vi "INTERLOCK SETTING.vi"() -> ()   [LabVIEW 2017]
uses:
  <vilib>/addons/database/Connection.llb/DB Tools Open Connec (Path).vi
  <vilib>/addons/_office/excel.llb/Excel Get Data ([str]).vi
  <vilib>/addons/_office/excel.llb/Excel Easy Table (str).vi
  <vilib>/Utility/NIReport.llb/NI_report.lvclass
  <vilib>/addons/database/NI_Database_API.lvlib
  <vilib>/addons/_office/NI_ReportGenerationToolkit.lvlib
  <vilib>/Utility/NIReport.llb/Excel/NI_Excel.lvclass
panel:
  in  "RECIPE PATH":path
  in  "EXPORT RECIPE":bool
  in  "Import Recipe":bool
  in  "table":string[][](table)
  in  "EXIT":bool
  in  "SAVE":bool
  # "PARAMETERS VALUE"
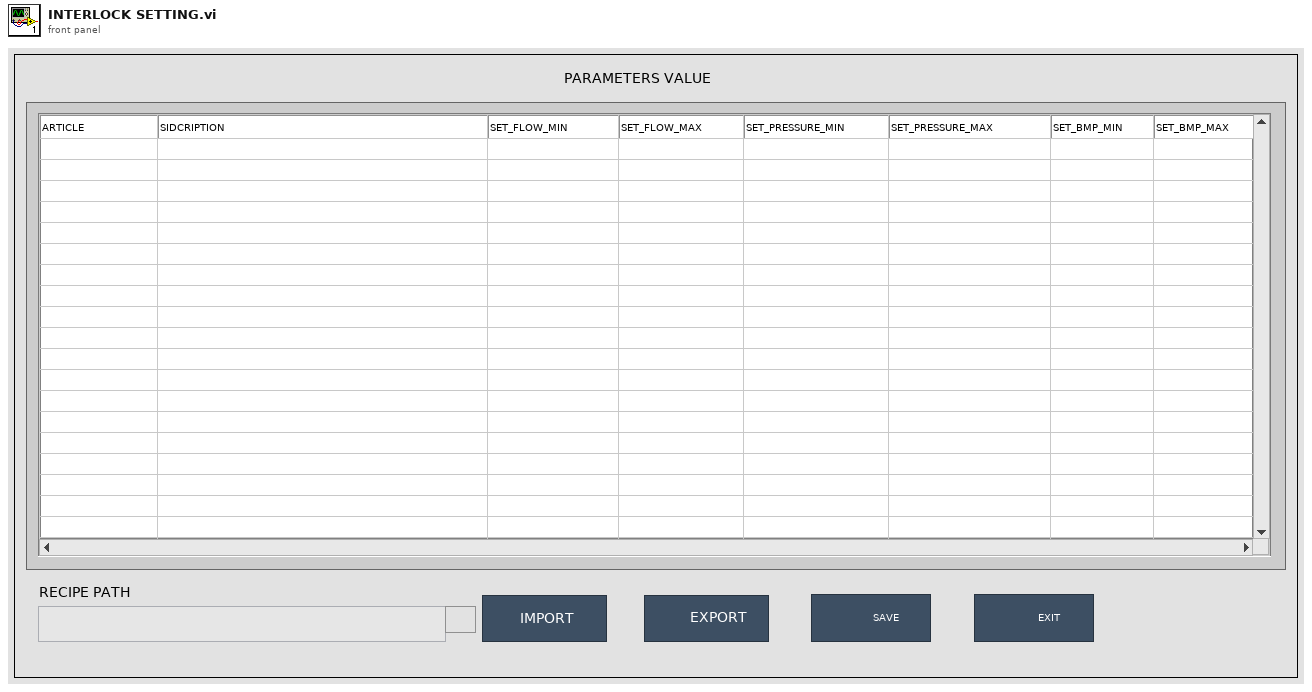
[diagram p1: front panel]
types:
  T1 = typedef "NI_Database_API.lvlib/Conn ObjectReference.ctl" = refnum<k1>
  T2 = enum16{"Standard Report", "HTML", "Word", "Excel"}
  T3 = enum16{"maximized", "minimized", "normal", "no change"}
  T4 = cluster{"table":string[], "table":string[], "table":string[], "table":string[], "table":string[], "table":string[], "table":string[], "table":string[]}
  T5 = enum32{"invalid app kind", "Development System", "Run Time System", "Student Edition", "Embedded LabVIEW", "Evaluation", "Custom"}
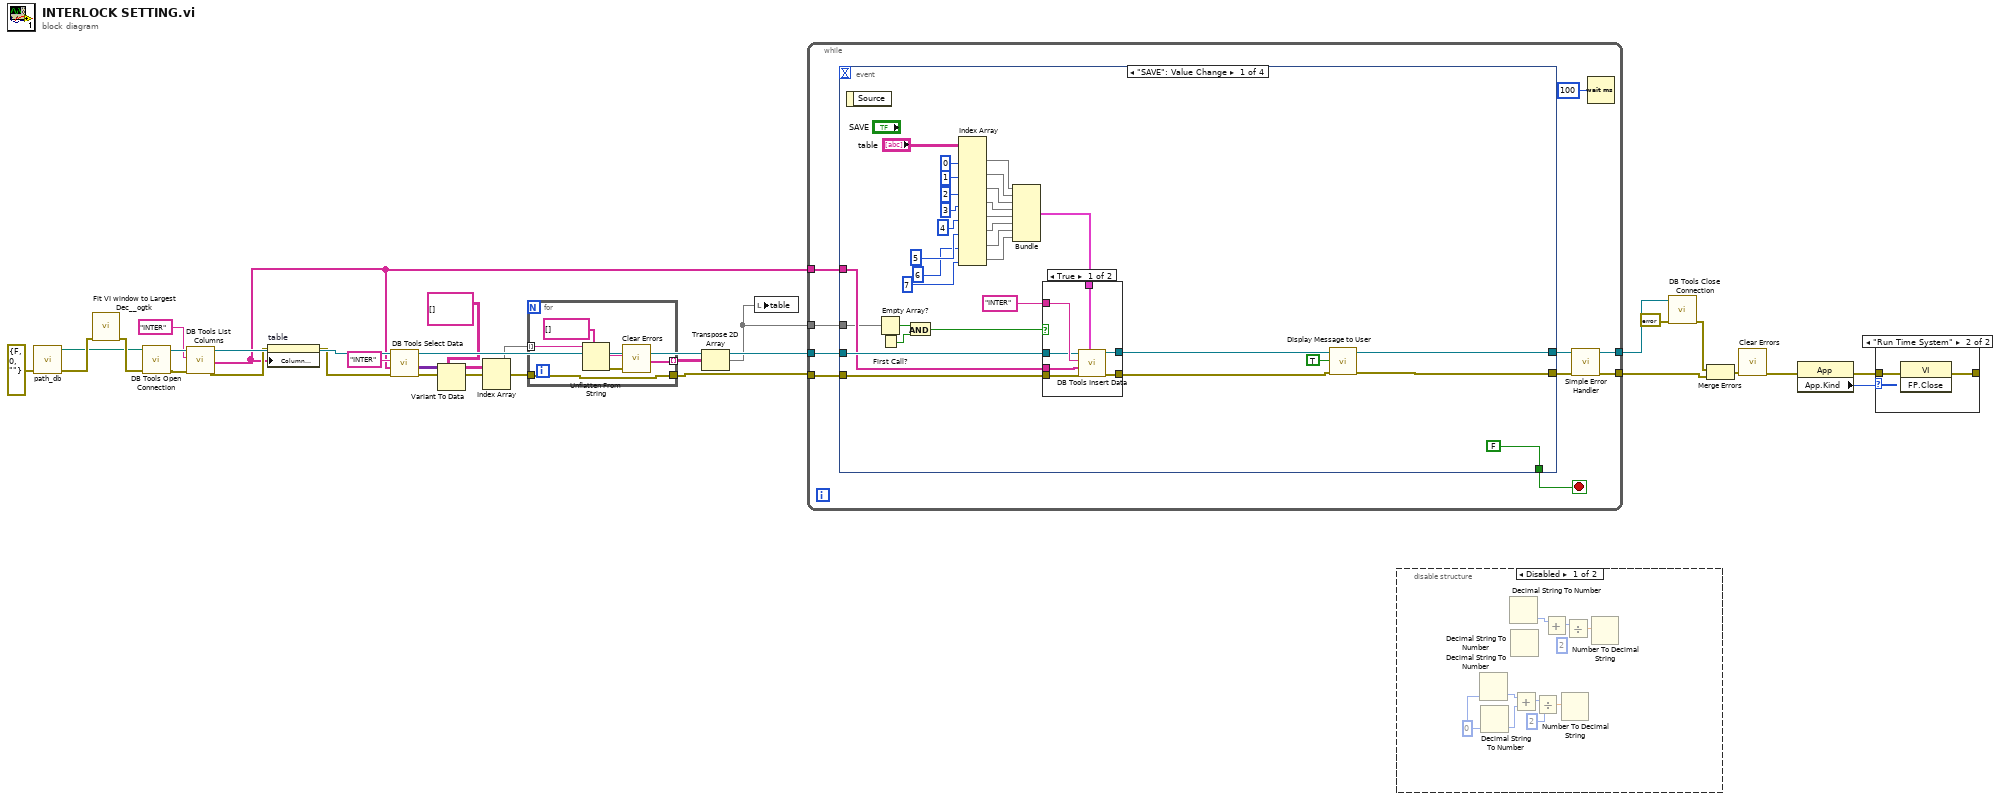
[diagram p0: block diagram]
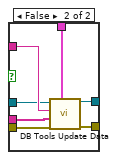
[diagram p4: hidden frame]
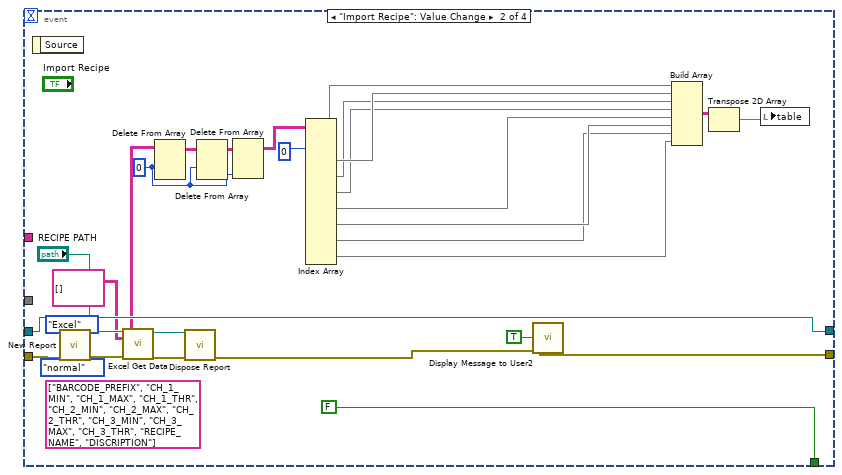
[diagram p5: hidden frame]
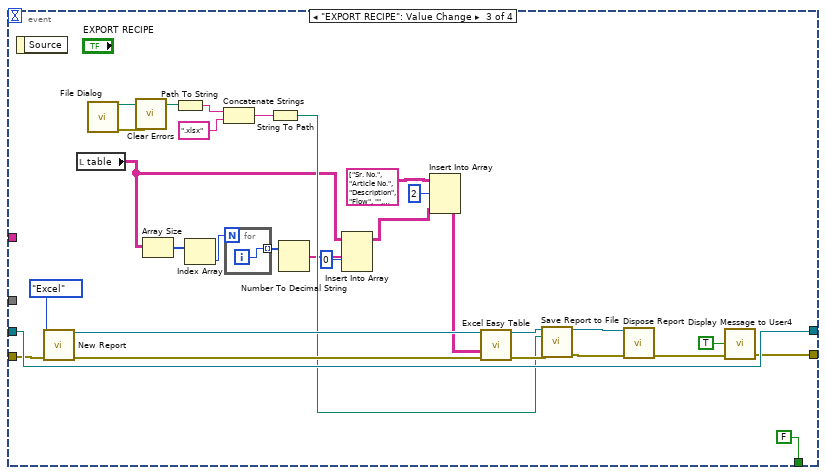
[diagram p6: hidden frame]
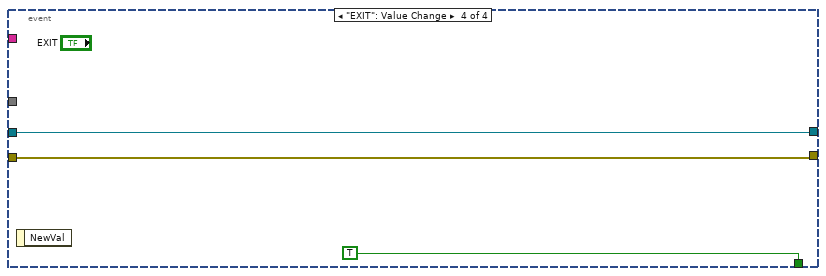
[diagram p7: hidden frame]
diagram:
  n1 = call "path_db.vi"("error in"=errorcluster {"status"=FALSE, "code"=0, "source"=""}) -> ("error out"=w17:errorcluster, "resulting string"=w8:path)  [unwired: 9 in]
  n2 = call <userlib>:"Fit VI window to Largest Dec__ogtk.vi"("error in (no error)"=w17) -> ("error out"=w16:errorcluster)  [unwired: 5 in, 1 out]
  n3 = call-poly <vilib>:"DB Tools Open Connection.vi"("error in (no error)"=w16, "connection information"=w8) -> ("error out"=w14:errorcluster, "connection reference"=w13:T1)  [unwired: 6 in]
  n4 = call <vilib>:"DB Tools List Columns.vi"("error in (no error)"=w14, "table"="INTER", "connection reference"=w13) -> ("error out"=w10:errorcluster, "columns"=w6:string[], "connection reference out"=w12:T1)  [unwired: 1 in, 1 out]
  n5 = property on="table" class="Tbl (strict)"(error in=w10, "Column Headers[]"=w6) -> (error out=w9:errorcluster)  [unwired: 1 in, 1 out]
  n6 = call <vilib>:"DB Tools Select Data.vi"("error in (no error)"=w9, "columns"=w6, "table"="INTER", "connection reference"=w12) -> ("error out"=w19:errorcluster, "data"=w23:variant[][], "connection reference out"=w26:T1)  [unwired: 2 in]
  n7 = Variant To Data(type=string[][] [], Variant=w23) -> (data=w22:string[][])  [unwired: 1 in, 1 out]
  n8 = Index Array(array=w22) -> (element=w21:string[])  [unwired: 2 in]
  n9 = for {
    tunnel: w21 -> [w33] mode=indexing
    tunnel: [w31] -> w20 mode=indexing
    tunnel: w19 -> [w30]
    tunnel: [w30] -> w18
    n10 = Unflatten From String(type=string[] [], binary string=w33) -> (value=w31:string[], error out=w34:errorcluster)  [unwired: 3 in, 1 out]
    n11 = call <vilib>:"Clear Errors.vi"("error in (no error)"=w34) -> ()  [unwired: 5 in, 2 out]
  }
  n12 = Transpose 2D Array(2D array=w20) -> (transposed array=w1:string[][])
  n13 = local write "table"(w1) -> ()
  n14 = while {
    tunnel: w18 -> [w42]
    tunnel: w26 -> [w41]
    tunnel: [w40] -> w29
    tunnel: [w38] -> w3
    tunnel: w6 -> [w36]
    tunnel: w1 -> [w35]
    stop <- w43 stop-if-true
    n15 = event shown="[0] \"SAVE\": Value Change" {
      selector: _ -> [_ _ _ _]
      dyn-events: _ -> [_ _ _ _]
      timeout: _ -> [_ _ _ _]
      tunnel: [FALSE FALSE FALSE TRUE] -> w43
      tunnel: w42 -> [w72 w106 w142 w149]
      tunnel: w41 -> [w71 w117 w146 w150]
      tunnel: [w70 w117 w146 w150] -> w40
      tunnel: [w50 w116 w145 w149] -> w39
      tunnel: w36 -> [w48 _ _ _]
      tunnel: w35 -> [w47 _ _ _]
      event "SAVE": Value Change {
        n16 = event-data() -> ()  [unwired: 1 in, 1 out]
        n17 = Empty Array?(array=w47) -> (empty?=w46:bool)
        n18 = First Call?() -> (First Call?: T/F=w45:bool)
        n19 = And(x=w46, y=w45) -> (x .and. y?=w44:bool)
        n20 = Index Array(array="table", index (col) #1=0 ("disabled index (col)"), index (col) #2=1 ("index (col)"), index (col) #3=2 ("index (col)"), index (col) #4=3 ("index (col)"), index (col) #5=4 ("index (col)"), index (col) #6=5 ("index (col)"), index (col) #7=6 ("index (col)"), index (col) #8=7 ("index (col)")) -> (element #1=w64:string[], element #2=w61:string[], element #3=w62:string[], element #4=w63:string[], element #5=w55:string[], element #6=w54:string[], element #7=w53:string[], element #8=w52:string[])  [unwired: 8 in]
        n21 = Bundle("table"=w64, "table"=w61, "table"=w62, "table"=w63, "table"=w55, "table"=w54, "table"=w53, "table"=w52) -> (w60:T4)  [unwired: 1 in]
        n22 = case shown="True" w44 {
          tunnel: "INTER" ("table") -> [w81 w88]
          tunnel: w72 -> [w80 w87]
          tunnel: w71 -> [w79 w86]
          tunnel: [w78 w85] -> w70
          tunnel: w60 -> [w77 w84]
          tunnel: [w76 w83] -> w51
          tunnel: w48 -> [w75 w82]
          frame True {
            n23 = call <vilib>:"DB Tools Insert Data.vi"("data"=w77, "error in (no error)"=w80, "columns"=w75, "table"=w81, "connection reference"=w79) -> ("error out"=w76:errorcluster, "connection reference out"=w78:T1)  [unwired: 5 in]
          }
          frame False {
            n24 = call <vilib>:"DB Tools Update Data.vi"("data"=w84, "error in (no error)"=w87, "columns"=w82, "table"=w88, "connection reference"=w86) -> ("error out"=w83:errorcluster, "connection reference out"=w85:T1)  [unwired: 5 in]
          }
        }
        n25 = call "Display Message to User"("error in (no error)"=w51, "Enable"=TRUE) -> ("error out"=w50:errorcluster)  [unwired: 8 in, 1 out]
      }
      event "Import Recipe": Value Change {
        w102 = 0 ("index (row)")
        (unwired) string[] ["BARCODE_PREFIX", "CH_1_MIN", "CH_1_MAX", "CH_1_THR", "CH_2_MIN", "CH_2_MAX", "CH_2_THR", "CH_3_MIN", "CH_3_MAX", "CH_3_THR", "RECIPE_NAME", "DISCRIPTION"]
        n26 = event-data() -> ()  [unwired: 1 in, 1 out]
        n27 = call <vilib>:"New Report.vi"("window state (normal)"=T3."normal", "report type"=T2."Excel", "template (empty)"="RECIPE PATH", "error in (no error)"=w106) -> ("report out"=w109:refnum<class "NI_report.lvclass">, "error out"=w110:errorcluster)  [unwired: 10 in]
        n28 = call-poly <vilib>:"Excel Get Data.vi"("report in"=w109, "data type"=string[][] [], "error in (no error)"=w110) -> ("report out"=w111:refnum<class "NI_report.lvclass">, "data"=w89:string[][], "error out"=w112:errorcluster)  [unwired: 10 in]
        n29 = Delete From Array(array=w89, index (row)=w102) -> (array with subset deleted=w104:string[][])  [unwired: 2 in, 1 out]
        n30 = call-dynamic "Dispose Report.vi"("report in"=w111, "error in (no error)"=w112) -> ("error out"=w105:errorcluster)  [unwired: 13 in]
        n31 = Delete From Array(array=w104, index (row)=w102) -> (array with subset deleted=w103:string[][])  [unwired: 2 in, 1 out]
        n32 = Delete From Array(array=w103, index (col)=w102) -> (array with subset deleted=w101:string[][])  [unwired: 2 in, 1 out]
        n33 = Index Array(array=w101, index (col) #1=0 ("disabled index (col)")) -> (element #1=w99:string[], element #2=w98:string[], element #3=w95:string[], element #4=w94:string[], element #5=w93:string[], element #6=w92:string[], element #7=w91:string[], element #8=w90:string[])  [unwired: 15 in]
        n34 = call "Display Message to User2"("error in (no error)"=w105, "Enable"=TRUE) -> ("error out"=w116:errorcluster)  [unwired: 8 in, 1 out]
        n35 = Build Array(w99, w98, w95, w94, w93, w92, w91, w90) -> (w97:string[][])
        n36 = Transpose 2D Array(2D array=w97) -> (transposed array=w96:string[][])
        n37 = local write "table"(w96) -> ()
      }
      event "EXPORT RECIPE": Value Change {
        n38 = event-data() -> ()  [unwired: 1 in, 1 out]
        n39 = call <vilib>:"New Report.vi"("report type"=T2."Excel", "error in (no error)"=w142) -> ("report out"=w134:refnum<class "NI_report.lvclass">, "error out"=w135:errorcluster)  [unwired: 12 in]
        n40 = local read "table"() -> (w120:string[][])
        n41 = call "File Dialog"() -> ("selected path"=w136:path, "error out"=w140:errorcluster)  [unwired: 12 in, 2 out]
        n42 = call <vilib>:"Clear Errors.vi"("error in (no error)"=w140) -> ()  [unwired: 5 in, 2 out]
        n43 = Array Size(array=w120) -> (size(s)=w128:i32[])
        n44 = Path To String(path=w136) -> (string=w137:string)
        n45 = Index Array(array=w128) -> (element=w127:i32)  [unwired: 1 in]
        n46 = Concatenate Strings(w137, ".xlsx" ("string")) -> (w139:string)
        n47 = for {
          N: w127 -> [_]
          tunnel: [w148] -> w126 mode=indexing
          i -> [w148]
        }
        n48 = String To Path(string=w139) -> (path=w129:path)
        n49 = Number To Decimal String(number=w126) -> (decimal integer string=w125:string[])  [unwired: 1 in]
        n50 = Insert Into Array(array=w120, index (col)=0 ("disabled index (col)"), new element=w125) -> (w124:string[][])  [unwired: 1 in]
        n51 = Insert Into Array(array=string[][] [["Sr. No.", "Article No.", "Description", "Flow", "", "Pressure", "", "BPM", ""], ["", "", "", "Min", "Max", "Min", "Max", "Min", "Max"]] ("appended array"), index (row)=2, new element=w124) -> (w119:string[][])  [unwired: 1 in]
        n52 = call-poly <vilib>:"Excel Easy Table.vi"("report in"=w134, "text data"=w119, "error in (no error)"=w135) -> ("report out"=w131:refnum<class "NI_report.lvclass">, "error out"=w133:errorcluster)  [unwired: 8 in, 3 out]
        n53 = call-dynamic "Save Report to File.vi"("report in"=w131, "report file path"=w129, "error in (no error)"=w133) -> ("report out"=w130:refnum<class "NI_report.lvclass">, "error out"=w132:errorcluster)  [unwired: 11 in]
        n54 = call-dynamic "Dispose Report.vi"("report in"=w130, "error in (no error)"=w132) -> ("error out"=w141:errorcluster)  [unwired: 13 in]
        n55 = call "Display Message to User4"("error in (no error)"=w141, "Enable"=TRUE) -> ("error out"=w145:errorcluster)  [unwired: 8 in, 1 out]
      }
      event "EXIT": Value Change {
        n56 = event-data() -> ()  [unwired: 1 in, 1 out]
      }
    }
    n57 = call <vilib>:"Simple Error Handler.vi"("error in (no error)"=w39) -> ("error out"=w38:errorcluster)  [unwired: 4 in, 4 out]
    n58 = Wait (ms)(milliseconds to wait=u32 100) -> ()  [unwired: 1 out]
  }
  n59 = disable-structure shown="Disabled" {
    frame Disabled {
      (unwired) 2
      w155 = u64 0 ("default (0 I32)")
      n60 = Decimal String To Number(default (0L)=w155) -> (number=w157:u64)  [unwired: 2 in, 1 out]
      n61 = Decimal String To Number(default (0L)=w155) -> (number=w158:u64)  [unwired: 2 in, 1 out]
      n62 = Decimal String To Number() -> (number=w154:i32)  [unwired: 3 in, 1 out]
      n63 = Decimal String To Number() -> ()  [unwired: 3 in, 2 out]
      n64 = Add(x=w157, y=w158) -> (x+y=w159:u64)
      n65 = Divide(x=w159, y=2) -> (x/y=w160:dbl)
      n66 = Add(x=w154) -> (x+y=w153:i32)  [unwired: 1 in]
      n67 = Number To Decimal String(number=w160) -> ()  [unwired: 1 in, 1 out]
      n68 = Divide(x=w153) -> (x/y=w152:dbl)  [unwired: 1 in]
      n69 = Number To Decimal String(number=w152) -> ()  [unwired: 1 in, 1 out]
    }
    frame Enabled {
    }
  }
  n70 = call <vilib>:"DB Tools Close Connection.vi"("error in (no error)"=errorcluster {"status"=FALSE, "code"=0, "source"=""}, "connection reference"=w29) -> ("error out"=w4:errorcluster)  [unwired: 5 in]
  n71 = Merge Errors(w4, w3) -> (w2:errorcluster)
  n72 = call <vilib>:"Clear Errors.vi"("error in (no error)"=w2) -> ("error out"=w7:errorcluster)  [unwired: 5 in, 1 out]
  n73 = property class="App"(error in=w7) -> (error out=w27:errorcluster, "App.Kind"=w28:T5)  [unwired: 1 in, 1 out]
  n74 = case shown="\"Run Time System\"" w28 {
    tunnel: w27 -> [w161 w163]
    tunnel: [w161 w162] -> _
    frame Default {
    }
    frame "Run Time System" {
      n75 = invoke class="VI" method="FP.Close"(error in=w163) -> (error out=w162:errorcluster)  [unwired: 2 in, 2 out]
    }
  }
